vi "Enqueue Read-ON.vi"(8 "Error In":errorcluster, 9 "Waitting Time (s)":u8=20, 10 "Storage Zone":u8=20, 11 "Name":string) -> (0 "Error Out":errorcluster, 2 "Data":variant)   [LabVIEW 2019, in "SR_2000.lvlib"]
uses:
  SR_2000.lvlib
  Queue/Queue.lvlib
  Data Error Notifier/Data and Error Notifier.lvlib
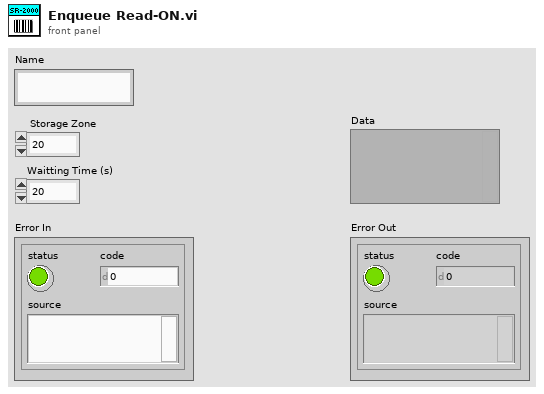
[diagram p1: front panel]
types:
  T1 = cluster{"Waitting Time (s)":u8, "Àx¦s°Ï(1~16)":u8}
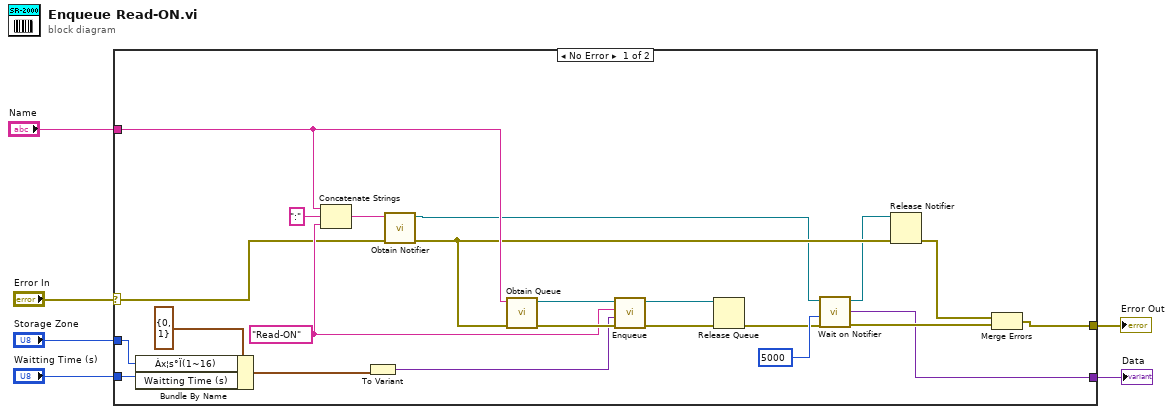
[diagram p0: block diagram]
diagram:
  n1 = case shown="No Error" "Error In" {
    selector: "Error In" -> [w18 w30]
    tunnel: [w21 w30] -> w5
    tunnel: "Name" -> [w28 _]
    tunnel: "Storage Zone" -> [w10 _]
    tunnel: [w11 _] -> w2
    tunnel: "Waitting Time (s)" -> [w9 _]
    frame No Error {
      w26 = "Read-ON" ("Message")
      n2 = Bundle By Name(cluster=T1 {"Waitting Time (s)"=0, "Àx¦s°Ï(1~16)"=1}, "Àx¦s°Ï(1~16)"=w10, "Waitting Time (s)"=w9) -> (w7:T1)
      n3 = Concatenate Strings(w28, ":" ("string"), w26) -> (w19:string)
      n4 = To Variant(anything=w7) -> (Variant=w20:variant)
      n5 = call "Obtain Notifier.vi"("Error In"=w18, "Name"=w19) -> ("Error Out"=w17:errorcluster, "notifier out"=w16:refnum<notifier>)  [unwired: 8 in]
      n6 = call "Obtain Queue.vi"("Error In"=w17, "Name"=w28) -> ("Error Out"=w29:errorcluster, "queue out"=w24:refnum<queue>)  [unwired: 8 in]
      n7 = call "Enqueue.vi"("Error In"=w29, "Data"=w20, "Message"=w26, "queue in"=w24) -> ("Error Out"=w25:errorcluster, "queue out"=w23:refnum<queue>)  [unwired: 6 in]
      n8 = Release Queue(queue=w23, error in (no error)=w25) -> (error out=w14:errorcluster)  [unwired: 1 in, 2 out]
      n9 = call "Wait on Notifier.vi"("Error In"=w14, "timeout in ms (-1)"=5000, "notifier in"=w16) -> ("Error Out"=w12:errorcluster, "Data"=w11:variant, "notifier out"=w13:refnum<notifier>)  [unwired: 6 in]
      n10 = Release Notifier(notifier=w13, error in (no error)=w17) -> (error out=w22:errorcluster)  [unwired: 1 in, 2 out]
      n11 = Merge Errors(w22, w12) -> (w21:errorcluster)
    }
    frame Error {
    }
  }
  "Error Out" <- w5
  "Data" <- w2
